vi "Calculate Dynamic Item Absolute Path.vi"(10 "Compat Built App Relative Path":path, 11 "Core Relative Path":path) -> (3 "Resulting Absolute Path":path)   [LabVIEW 2020, in "NI_ReportGenerationCore.lvlib"]
uses:
  <vilib>/Utility/NIReport.llb/NI_ReportGenerationCore.lvlib
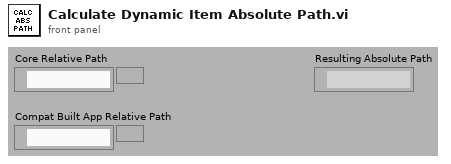
[diagram p1: front panel]
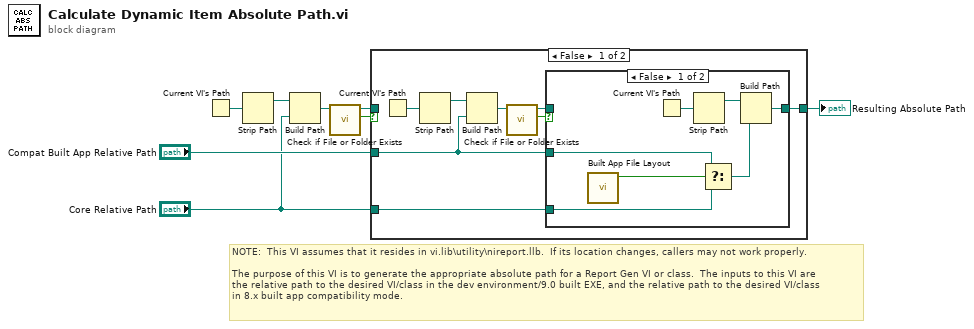
[diagram p0: block diagram]
diagram:
  # "NOTE:  This VI assumes that it resides in vi.lib\\utility\\nireport.llb.  If its location changes, callers may not work properly.\n\nThe purpose of this VI is to generate the appropriate absolute path for a Report Gen VI or class.  The inputs to this VI are\nthe relative path to the desired VI/class in the dev environment/9.0 built EXE, and the relative path to the desired VI/class\nin 8.x built app compatibility mode."
  n1 = Current VI's Path() -> (path=w3:path)
  n2 = Strip Path(path=w3) -> (stripped path=w2:path)  [unwired: 1 out]
  n3 = Build Path(base path=w2, name or relative path="Core Relative Path") -> (appended path=w4:path)
  n4 = call <vilib>:"Check if File or Folder Exists.vi"("path"=w4) -> ("file or folder exists?"=w5:bool, "dup path"=w6:path)  [unwired: 1 in, 8 out]
  n5 = case shown="False" w5 {
    tunnel: [w16 w25] -> w1
    tunnel: w6 -> [_ w25]
    tunnel: "Core Relative Path" -> [w10 _]
    tunnel: "Compat Built App Relative Path" -> [w9 _]
    frame False {
      n6 = Current VI's Path() -> (path=w14:path)
      n7 = Strip Path(path=w14) -> (stripped path=w13:path)  [unwired: 1 out]
      n8 = Build Path(base path=w13, name or relative path=w9) -> (appended path=w15:path)
      n9 = call <vilib>:"Check if File or Folder Exists.vi"("path"=w15) -> ("file or folder exists?"=w12:bool, "dup path"=w11:path)  [unwired: 1 in, 8 out]
      n10 = case shown="False" w12 {
        tunnel: [w21 w24] -> w16
        tunnel: w11 -> [_ w24]
        tunnel: w10 -> [w18 _]
        tunnel: w9 -> [w17 _]
        frame False {
          n11 = call <vilib>:"Built App File Layout.vi"() -> ("Legacy Layout?"=w19:bool)  [unwired: 1 in, 10 out]
          n12 = Current VI's Path() -> (path=w23:path)
          n13 = Strip Path(path=w23) -> (stripped path=w22:path)  [unwired: 1 out]
          n14 = Select(t=w17, s=w19, f=w18) -> (s? t:f=w20:path)
          n15 = Build Path(base path=w22, name or relative path=w20) -> (appended path=w21:path)
        }
        frame True {
        }
      }
    }
    frame True {
    }
  }
  "Resulting Absolute Path" <- w1
